vi "secondary.vi"() -> ()   [LabVIEW 2018]
uses:
  MotorController/#include/Global textParse.vi
panel:
  out "Vsense":bool
  out "VSense Measure":dbl
  in  "E-Stop":bool
  out "Vload":bool
  out "Vload Measure":dbl
  out "refnum out":refnum<file>
  in  "Number of Oscilloscopes":bool caption="Boolean"
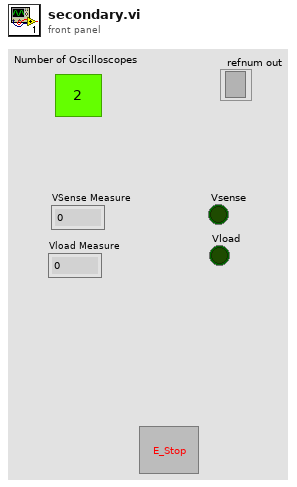
[diagram p1: front panel]
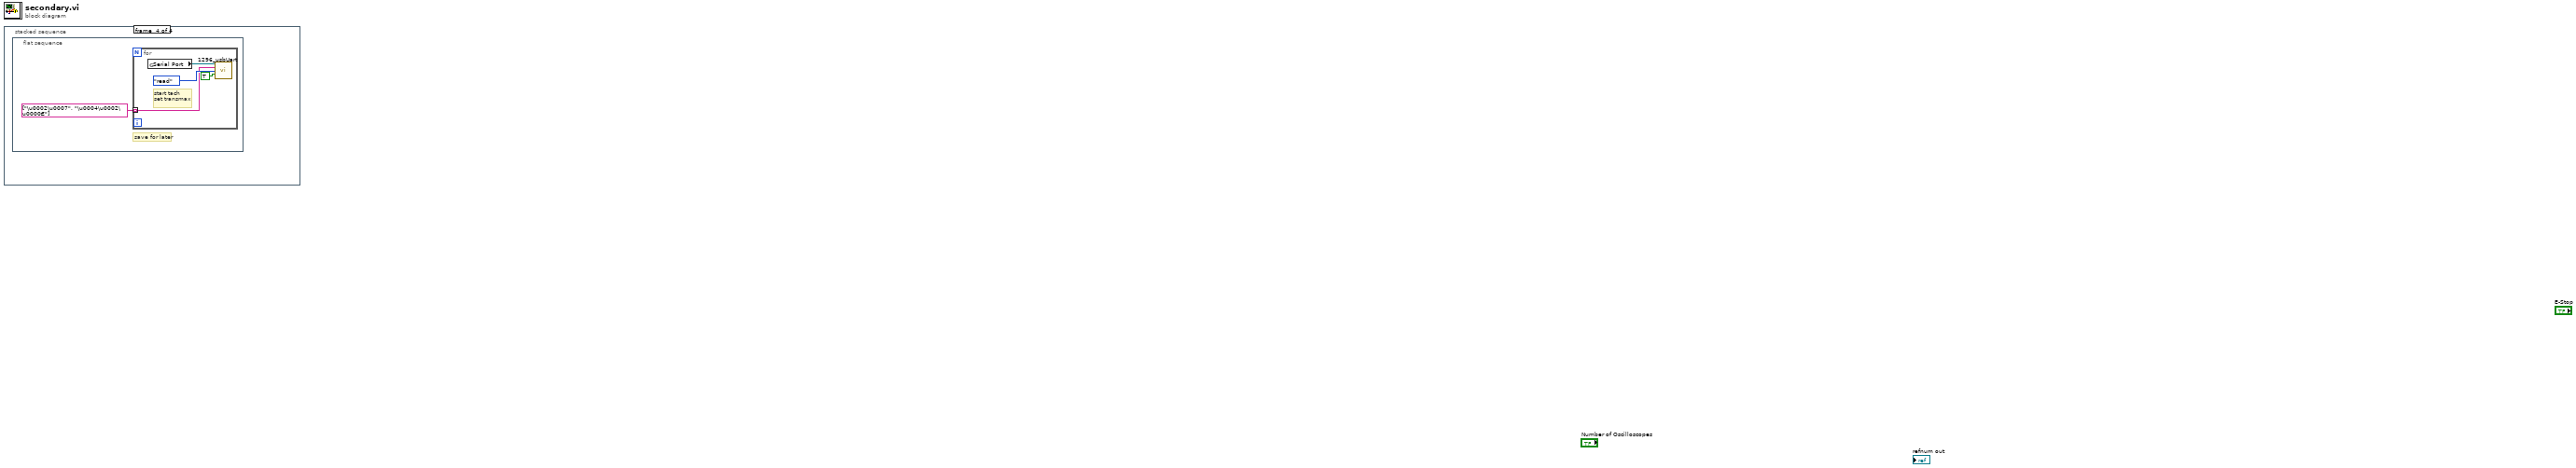
[diagram p0: block diagram]
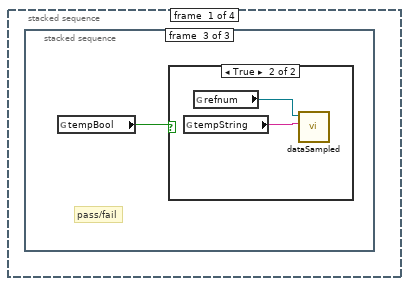
[diagram p2: hidden frame]
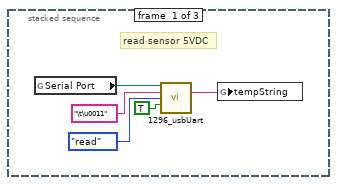
[diagram p3: hidden frame]
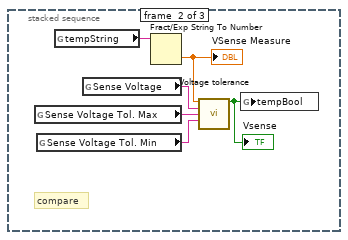
[diagram p4: hidden frame]
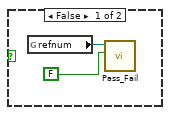
[diagram p5: hidden frame]
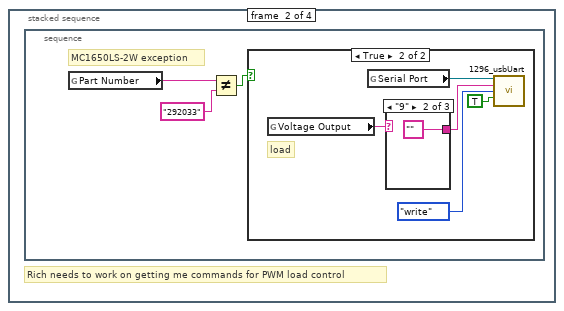
[diagram p6: hidden frame]
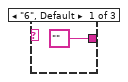
[diagram p8: hidden frame]
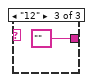
[diagram p9: hidden frame]
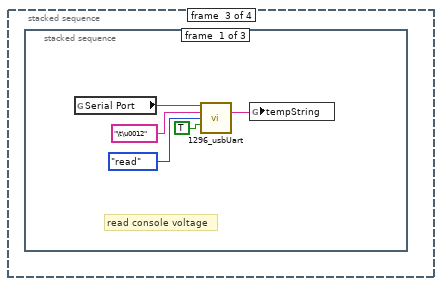
[diagram p10: hidden frame]
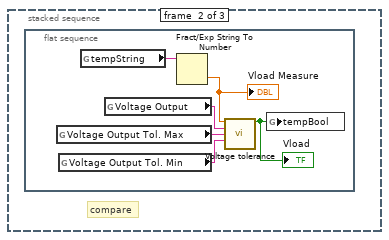
[diagram p11: hidden frame]
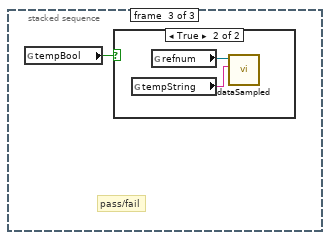
[diagram p12: hidden frame]
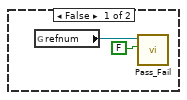
[diagram p13: hidden frame]
diagram:
  n1 = stacked-sequence {
    frame #0 {
      n2 = stacked-sequence {
        frame #0 {
          # "read sensor 5VDC"
          n3 = global read "Global textParse.vi" "Serial Port"() -> (w5:refnum<visa-resource-name>)
          n4 = call "1296_usbUart.vi"("VISA resource name"=w5, "command"="\t\u0011", "r/w"=enum16{"read", "write"}."read", "resetValues"=TRUE) -> ("byte[4]"=w1:string)  [unwired: 8 in, 3 out]
          n5 = global write "Global textParse.vi" "tempString"(w1) -> ()
        }
        frame #1 {
          # "compare"
          n6 = global read "Global textParse.vi" "Sense Voltage Tol. Max"() -> (w9:string)
          n7 = global read "Global textParse.vi" "Sense Voltage Tol. Min"() -> (w8:string)
          n8 = global read "Global textParse.vi" "tempString"() -> (w11:string)
          n9 = global read "Global textParse.vi" "Sense Voltage"() -> (w10:string)
          n10 = Fract/Exp String To Number(string=w11) -> (number=w7:dbl)  [unwired: 3 in, 1 out]
          "VSense Measure" <- w7
          n11 = call "Voltage tolerance.vi"("Data Sample"=w7, "Spec Output"=w10, "Upper"=w9, "Lower"=w8) -> ("Boolean"=w6:bool)  [unwired: 10 in, 1 out]
          "Vsense" <- w6
          n12 = global write "Global textParse.vi" "tempBool"(w6) -> ()
        }
        frame #2 {
          # "pass/fail"
          n13 = global read "Global textParse.vi" "tempBool"() -> (w12:bool)
          n14 = case shown="True" w12 {
            frame False {
              n15 = global read "Global textParse.vi" "refnum"() -> (w14:refnum<file>)
              n16 = call "Pass_Fail.vi"("OK"=FALSE, "Byte Stream File in"=w14) -> ()  [unwired: 8 in, 2 out]
            }
            frame True {
              n17 = global read "Global textParse.vi" "tempString"() -> (w16:string)
              n18 = global read "Global textParse.vi" "refnum"() -> (w15:refnum<file>)
              n19 = call "dataSampled.vi"("Data"=w16, "refnum in"=w15) -> ()  [unwired: 8 in, 2 out]
            }
          }
        }
      }
    }
    frame #1 {
      # "Rich needs to work on getting me commands for PWM load control"
      n20 = stacked-sequence {
        frame #0 {
          # "MC1650LS-2W exception"
          n21 = global read "Global textParse.vi" "Part Number"() -> (w18:string)
          n22 = Not Equal?(x=w18, y="292033") -> (x != y?=w17:bool)
          n23 = case shown="True" w17 {
            frame False {
              # "no load"
            }
            frame True {
              # "load"
              n24 = global read "Global textParse.vi" "Voltage Output"() -> (w24:string)
              n25 = global read "Global textParse.vi" "Serial Port"() -> (w23:refnum<visa-resource-name>)
              n26 = case shown="\"9\"" w24 {
                tunnel: ["" ("command") "" ("command") "" ("command")] -> w20
                frame "6", Default {
                }
                frame "9" {
                }
                frame "12" {
                }
              }
              n27 = call "1296_usbUart.vi"("VISA resource name"=w23, "command"=w20, "r/w"=enum16{"read", "write"}."write", "resetValues"=TRUE) -> ()  [unwired: 8 in, 4 out]
            }
          }
        }
      }
    }
    frame #2 {
      n28 = stacked-sequence {
        frame #0 {
          # "read console voltage"
          n29 = global read "Global textParse.vi" "Serial Port"() -> (w32:refnum<visa-resource-name>)
          n30 = call "1296_usbUart.vi"("VISA resource name"=w32, "command"="\t\u0012", "r/w"=enum16{"read", "write"}."read", "resetValues"=TRUE) -> ("byte[4]"=w28:string)  [unwired: 8 in, 3 out]
          n31 = global write "Global textParse.vi" "tempString"(w28) -> ()
        }
        frame #1 {
          # "compare"
          n32 = flat-sequence {
            frame #0 {
              n33 = global read "Global textParse.vi" "Voltage Output Tol. Max"() -> (w36:string)
              n34 = global read "Global textParse.vi" "Voltage Output Tol. Min"() -> (w35:string)
              n35 = global read "Global textParse.vi" "tempString"() -> (w38:string)
              n36 = global read "Global textParse.vi" "Voltage Output"() -> (w37:string)
              n37 = Fract/Exp String To Number(string=w38) -> (number=w33:dbl)  [unwired: 3 in, 1 out]
              "Vload Measure" <- w33
              n38 = call "Voltage tolerance.vi"("Data Sample"=w33, "Spec Output"=w37, "Upper"=w36, "Lower"=w35) -> ("Boolean"=w34:bool)  [unwired: 10 in, 1 out]
              "Vload" <- w34
              n39 = global write "Global textParse.vi" "tempBool"(w34) -> ()
            }
          }
        }
        frame #2 {
          # "pass/fail"
          n40 = global read "Global textParse.vi" "tempBool"() -> (w39:bool)
          n41 = case shown="True" w39 {
            frame False {
              n42 = global read "Global textParse.vi" "refnum"() -> (w41:refnum<file>)
              n43 = call "Pass_Fail.vi"("OK"=FALSE, "Byte Stream File in"=w41) -> ()  [unwired: 8 in, 2 out]
            }
            frame True {
              n44 = global read "Global textParse.vi" "tempString"() -> (w43:string)
              n45 = global read "Global textParse.vi" "refnum"() -> (w42:refnum<file>)
              n46 = call "dataSampled.vi"("Data"=w43, "refnum in"=w42) -> ()  [unwired: 8 in, 2 out]
            }
          }
        }
      }
    }
    frame #3 {
      n47 = flat-sequence {
        frame #0 {
          # "save for later"
          n48 = for {
            tunnel: string[] ["\u0002\u0007", "\u0004\u0002\u0000€"] -> [w45] mode=indexing
            # "start tach\nset transmax"
            n49 = global read "Global textParse.vi" "Serial Port"() -> (w48:refnum<visa-resource-name>)
            n50 = call "1296_usbUart.vi"("VISA resource name"=w48, "command"=w45, "r/w"=enum16{"read", "write"}."read", "resetValues"=TRUE) -> ()  [unwired: 8 in, 4 out]
          }
        }
      }
    }
  }
